vi "FrameRateWrite.vi"(4 "error in (no error)":errorcluster, 5 "Value":dbl, 6 "Container State":T4, 7 "Display State In":T1) -> (0 "error out":errorcluster, 3 "Display State Out":T1)   [LabVIEW 2013, in "AnimatorXControl.xctl"]
uses:
  AnimatorXControl.xctl
  <vilib>/_xctls/Container State.ctl
  AnimatorState.ctl
  <vilib>/picture/picture.llb/imagedata.ctl
  AnimatorSettings.ctl
  <vilib>/_xctls/XControlSupport.lvlib
panel:
  # "Replace the Value Control below with a Control of desired type.\nDo not remove this Control or the others from the connector pane.\nDo not change the connector pane pattern.\nThe Value control should always be the third terminal from top on the input side in the connector pane."
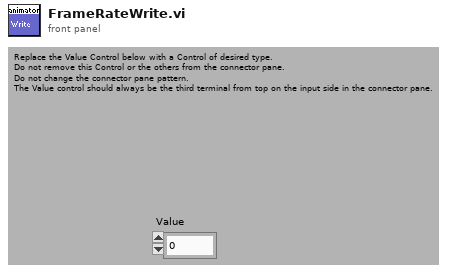
[diagram p1: front panel]
types:
  T1 = typedef "AnimatorXControl.xctl/AnimatorState.ctl" = cluster{"Images":cluster{"Files":path[], "ImageData":T2[]}, "Settings":T3}
  T2 = typedef "imagedata.ctl" = cluster{"image type":i32, "image depth":i32, "image":u8[], "mask":u8[], "colors":u32[], "Rectangle":cluster{"left":i16, "top":i16, "right":i16, "bottom":i16}}
  T3 = typedef "AnimatorXControl.xctl/AnimatorSettings.ctl" = cluster{"Reverse":bool, "FrameRate":dbl, "WorkMode":enum16{"Automatic", "UseValue"}}
  T4 = typedef "XControlSupport.lvlib/Container State.ctl" = cluster{"Indicator?":bool, "Run Mode?":bool, " Refnum":refnum<vi>}
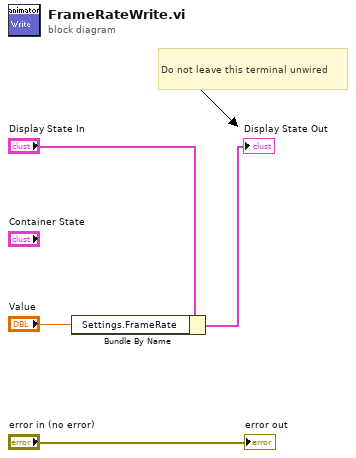
[diagram p0: block diagram]
diagram:
  # "Do not leave this terminal unwired"
  n1 = Bundle By Name(cluster="Display State In", "Settings.FrameRate"="Value") -> (→"Display State Out":T1)
  "error out" <- "error in (no error)"
